vi "InitMultiThermal.vi"(8 "error in":errorcluster, 10 "I2C Addresses":u8[](array[numeric]), 11 "LINX Resource in":T3) -> (0 "error out":errorcluster, 1 "ThermalConfigs":T1[](array[typedef]) {"Last Temp Readings"."Ambient Temp (°F)" format="%.2f °F"; "Last Temp Readings"."Ambient Temp (°C)" format="%.2f °C"; "Last Temp Readings"."Object Temp (°F)" format="%.2f °F"; "Last Temp Readings"."Object Temp (°C)" format="%.2f °C"; "Samples to Average" items=["1 sample, .26s conversion"=0, "2 samples, .51s conversion"=512, "4 samples, 1.01s conversion"=1024, "8 samples, 2.01s conversion"=1536, "16 samples, 4.01s conversion"=2048]; "I2C Slave Address" format="%.0x"}, 2 "ThermOnline":bool[](array[boolean]), 3 "LINX Resource out":T3)   [LabVIEW 2017]
uses:
  <vilib>/MakerHub/LINX/Private/Type Defs/Platform.ctl
  <vilib>/MakerHub/LINX/Private/Type Defs/Interface.ctl
  <vilib>/MakerHub/LINX/Private/Device/Type Defs/TCP Config.ctl
  <vilib>/MakerHub/LINX/Private/Device/Type Defs/Channels.ctl
  <vilib>/MakerHub/LINX/Private/Device/Type Defs/LINX Device Config.ctl
  <vilib>/MakerHub/LINX/Private/Type Defs/LINX Ref.ctl
  Type Defs/tempReadings.ctl
  Type Defs/thermopileSettings.ctl
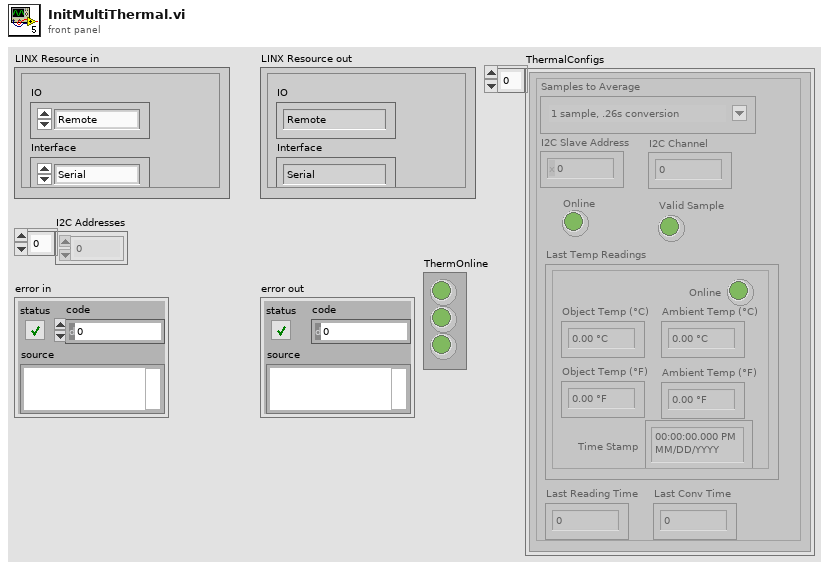
[diagram p1: front panel]
types:
  T1 = typedef "thermopileSettings.ctl" = cluster{"Online":bool, "I2C Channel":u8, "I2C Slave Address":u8, "Valid Sample":bool, "Samples to Average":u16, "Last Temp Readings":T2, "Last Reading Time":dbl, "Last Conv Time":dbl}
  T2 = typedef "tempReadings.ctl" = cluster{"Object Temp (°C)":dbl, "Object Temp (°F)":dbl, "Ambient Temp (°C)":dbl, "Ambient Temp (°F)":dbl, "Online":bool, "Time Stamp":timestamp}
  T3 = typedef "LMH-LINX.lvlib/LINX Ref.ctl" = cluster{"IO":T4, "Interface":T5, "LINX Device Config":T6}
  T4 = typedef "LMH-LINX.lvlib/Platform.ctl" = enum16{"Remote", "Local"}
  T5 = typedef "LMH-LINX.lvlib/Interface.ctl" = enum16{"Serial", "TCP"}
  T6 = typedef "LMH-LINX.lvlib/Device.lvlib/LINX Device Config.ctl" = cluster{"Interface":T5, "COM Port":refnum<visa-resource-name>, "TCP Configuration":T7, "Device Family":u8, "Device ID":u8, "Device Name":string, "TCP Ref":refnum<k5>, "Channels":T8}
  T7 = typedef "LMH-LINX.lvlib/Device.lvlib/TCP Config.ctl" = cluster{"IP Address":string, "Port":u16}
  T8 = typedef "LMH-LINX.lvlib/Channels.ctl" = cluster{"DI":u8[], "DO":u8[], "AI":u8[], "AO":u8[], "PWM":u8[], "QE":u8[], "UART":u8[], "I2C 2":u8[], "SPI":u8[], "CAN":u8[], "Servo":u8[], "AI Ref (V)":dbl, "AI Resolution (Bits)":u8, "AO Ref (V)":dbl, "AO Resolution (Bits)":u8}
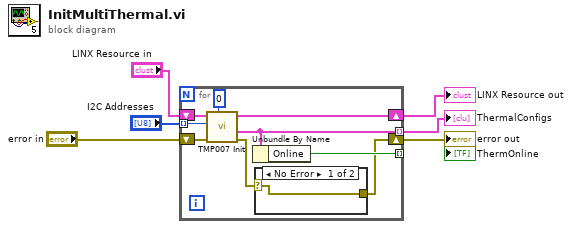
[diagram p0: block diagram]
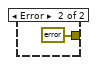
[diagram p2: hidden frame]
diagram:
  n1 = for {
    shift-right: [w8] -> w3
    shift-left: "error in" -> [w15]
    shift-right: [w13] -> w5
    shift-left: "LINX Resource in" -> [w14]
    tunnel: "I2C Addresses" -> [w12] mode=indexing
    tunnel: [w10] -> _ mode=indexing
    tunnel: [w7] -> w2 mode=indexing
    n2 = call "TMP007 Init.vi"("I2C Channel"=u8 0, "error in (no error)"=w15, "I2C Slave Address"=w12, "LINX Resource in"=w14) -> ("error out"=w9:errorcluster, "Thermopile Setting"=w7:T1, "LINX Resource out"=w13:T3)  [unwired: 5 in]
    n3 = Unbundle By Name(w7) -> ("Online"=w10:bool)
    n4 = case shown="No Error" w9 {
      selector: w9 -> [w16 _]
      tunnel: [w16 errorcluster {"status"=FALSE, "code"=0, "source"=""} ("error in 2")] -> w8
      frame No Error {
      }
      frame Error {
      }
    }
  }
  "LINX Resource out" <- w5
  "error out" <- w3
  "ThermalConfigs" <- w2
